vi "Graph Scroll Demo.vi"() -> ()   [LabVIEW 2022 SP3] (continued)
-40.6327, -40.053177, -40.0813, -40.27929, -40.53585, -40.08412, -39.742516, -40.55218, -40.517155, -40.038376, -40.539658, -39.79699, -40.197483, -40.014664, -39.99154, -40.9734, -40.019516, -40.305576, -40.771317, -40.490135, -40.648216, -40.34266, -40.4466, -40.38034, -40.224007, -40.007706, -39.885803, -40.199375, -40.56833, -40.193268, -40.08329, -40.476387, -41.044292, -41.039032, -40.65704, -40.33447, -40.63921, -40.425865]}, {"x0"=4.9754999999999994e-05, "dx"=4e-10, "y"=[-40.112347, -40.4553, -40.08172, -40.58159, -40.238785, -40.08866, -40.117218, -40.209885, -39.905983, -39.701725, -40.28698, -40.62065, -40.520744, -39.86386, -40.370846, -40.32646, -40.940292, -39.999413, -40.183598, -40.38126, -40.079338, -40.333084, -39.9855, -40.593704, -39.891304, -40.685226, -40.63095, -40.199932, -40.06239, -39.907475, -40.674614, -40.390415, -40.288296, -40.289345, -40.496902, -40.03651, -40.580055, -40.441357, -39.800877, -40.357933, -40.486122, -40.08663, -40.230988, -40.14924, -40.174007, -40.536613, -40.042187, -40.583797, -40.057236, -39.992195, -39.96219, -40.309696, -40.49513, -40.251595, -40.865784, -39.574238, -40.167404, -40.291233, -40.004013, -40.557858, -39.800873, -40.406208, -40.0242]}, {"x0"=4.9804999999999995e-05, "dx"=4e-10, "y"=[-40.30662, -40.336685, -39.80644, -39.773655, -40.124554, -40.164036, -40.05616, -40.427773, -39.873405, -40.580826, -40.20838, -40.017136, -40.620667, -39.976677, -40.97496, -39.8172, -40.038223, -40.150547, -40.289112, -40.23432, -40.495758, -40.797295, -40.08434, -39.72016, -39.82246, -40.110863, -39.75662, -39.894024, -40.69976, -40.332302, -39.80183, -40.044945, -40.382618, -40.62515, -40.415936, -39.86055, -39.952003, -40.133392, -39.95831, -40.171513, -40.75497, -39.738483, -40.02381, -40.737907, -39.95378, -40.15747, -40.33146, -40.07541, -40.187897, -40.130882, -40.588013, -40.471916, -40.171486, -40.30863, -40.275925, -40.40497, -39.72168, -40.562958, -40.443184, -40.50091, -40.94509, -40.832333, -40.25718]}, {"x0"=4.9854999999999996e-05, "dx"=4e-10, "y"=[-39.95831, -40.608727, -40.40875, -39.968494, -40.38857, -40.757965, -39.90829, -40.068916, -40.80175, -40.437004, -40.359303, -40.27329, -40.87732, -40.408707, -40.810448, -40.472916, -40.164375, -39.95311, -39.658043, -40.621872, -40.868988, -40.879944, -40.226665, -40.37654, -40.824974, -40.433846, -40.64727, -40.374466, -40.03051, -40.317833, -40.07064, -40.217545, -40.632515, -40.18609, -40.415688, -40.680775, -40.394157, -40.643803, -40.44794, -40.176754, -40.133392, -40.31482, -40.14257, -40.437088, -39.792526, -40.132427, -40.4438, -40.378223, -40.03153, -40.807022, -40.47294, -40.523907, -40.723423, -40.19915, -40.654327, -39.873405, -40.11151, -39.791588, -40.4874, -40.206738, -39.947983, -40.599842, -40.285004]}, {"x0"=4.9905e-05, "dx"=4e-10, "y"=[-40.635777, -40.429264, -40.221474, -40.53879, -40.084232, -40.543945, -40.09342, -40.699425, -40.281723, -40.349842, -40.965515, -40.19594, -40.393257, -40.991196, -40.167015, -40.089092, -40.28145, -40.1708, -40.1926, -40.168953, -40.216183, -40.054413, -40.477978, -40.311504, -40.105743, -40.781967, -40.03868, -39.941833, -40.212257, -40.22416, -40.465065, -40.427773, -40.041557, -40.30243, -40.076145, -40.384693, -41.042843, -40.60782, -40.46398, -40.251957, -40.58636, -40.241493, -40.23226, -39.859276, -40.34781, -40.84056, -40.268444, -40.38235, -40.25984, -40.302094, -40.49449, -39.87678, -40.723667, -40.34536, -40.065693, -41.03678, -40.669098, -40.325848, -40.158634, -40.184532, -40.35442, -40.120434, -40.631584]}, {"x0"=4.995499999999999e-05, "dx"=4e-10, "y"=[-39.93744, -40.200787, -40.19159, -40.312996, -40.304035, -40.026356, -40.159317, -40.17794, -40.507317, -40.75594, -40.2128, -40.69222, -40.509018, -40.132885, -40.38221, -40.535625, -40.671265, -40.074425, -40.66465, -40.046677, -40.04391, -40.59238, -40.578648, -40.728935, -40.355152, -40.12415, -40.326622, -40.20231, -40.076756, -40.34694, -40.473667, -40.44674, -40.506596, -40.33064, -39.931225, -40.38449, -39.91561, -39.918514, -40.172543, -40.180313, -40.2059, -40.21259, -40.28431, -40.623684, -39.96515, -40.036716, -40.128674, -40.348873, -40.544796, -40.175167, -40.266956, -40.36264, -39.99362, -40.116356, -40.16766, -40.155838, -40.825928, -40.394333, -39.406624, -40.61374, -40.241642, -40.76946]}] ("Amplitude (dBm) 2")
